vi "ClearFaults.vi"(11 "PM_Group in":refnum<class "PM_Group.lvclass">) -> (3 "PM_Group out":refnum<class "PM_Group.lvclass">)   [LabVIEW 2019, in "PM_Group.lvclass"]
uses:
  PM_Group.lvclass
  PM_Group.lvclass/PM_Group.ctl
  Engine_1DO_2DI_class/Engine_1DO_2DI.lvclass
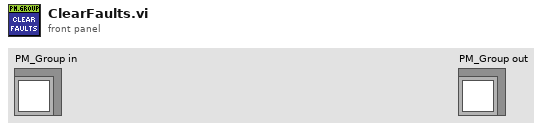
[diagram p1: front panel]
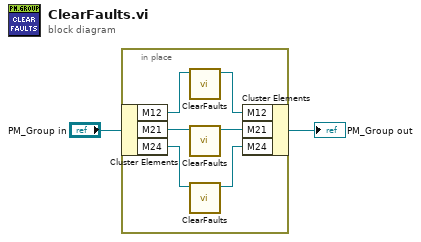
[diagram p0: block diagram]
diagram:
  n1 = in-place {
    n2 = in-place-cluster #1("PM_Group in") -> ("M12"=w8:refnum<class "Engine_1DO_2DI.lvclass">, "M21"=w6:refnum<class "Engine_1DO_2DI.lvclass">, "M24"=w5:refnum<class "Engine_1DO_2DI.lvclass">)
    n3 = call-dynamic "ClearFaults.vi"("Engine_1DO_2DI in"=w8) -> ("Engine_1DO_2DI out"=w7:refnum<class "Engine_1DO_2DI.lvclass">)  [unwired: 10 in]
    n4 = call-dynamic "ClearFaults.vi"("Engine_1DO_2DI in"=w6) -> ("Engine_1DO_2DI out"=w3:refnum<class "Engine_1DO_2DI.lvclass">)  [unwired: 10 in]
    n5 = call-dynamic "ClearFaults.vi"("Engine_1DO_2DI in"=w5) -> ("Engine_1DO_2DI out"=w4:refnum<class "Engine_1DO_2DI.lvclass">)  [unwired: 10 in]
    n6 = in-place-cluster #1("M12"=w7, "M21"=w3, "M24"=w4) -> (→"PM_Group out":refnum<class "PM_Group.lvclass">)
  }
